vi "CRYAPI TAB.vi"(8 "tPage":T1, 9 "tFrame":T3, 10 "nData":i32, 11 "sAction":string) -> (0 "nData_Out":i32, 2 "tFrame_Out":T3, 3 "tPage_Out":T1)   [LabVIEW 2013]
uses:
  <vilib>/Utility/miscctls.llb/LVRectTypeDef.ctl
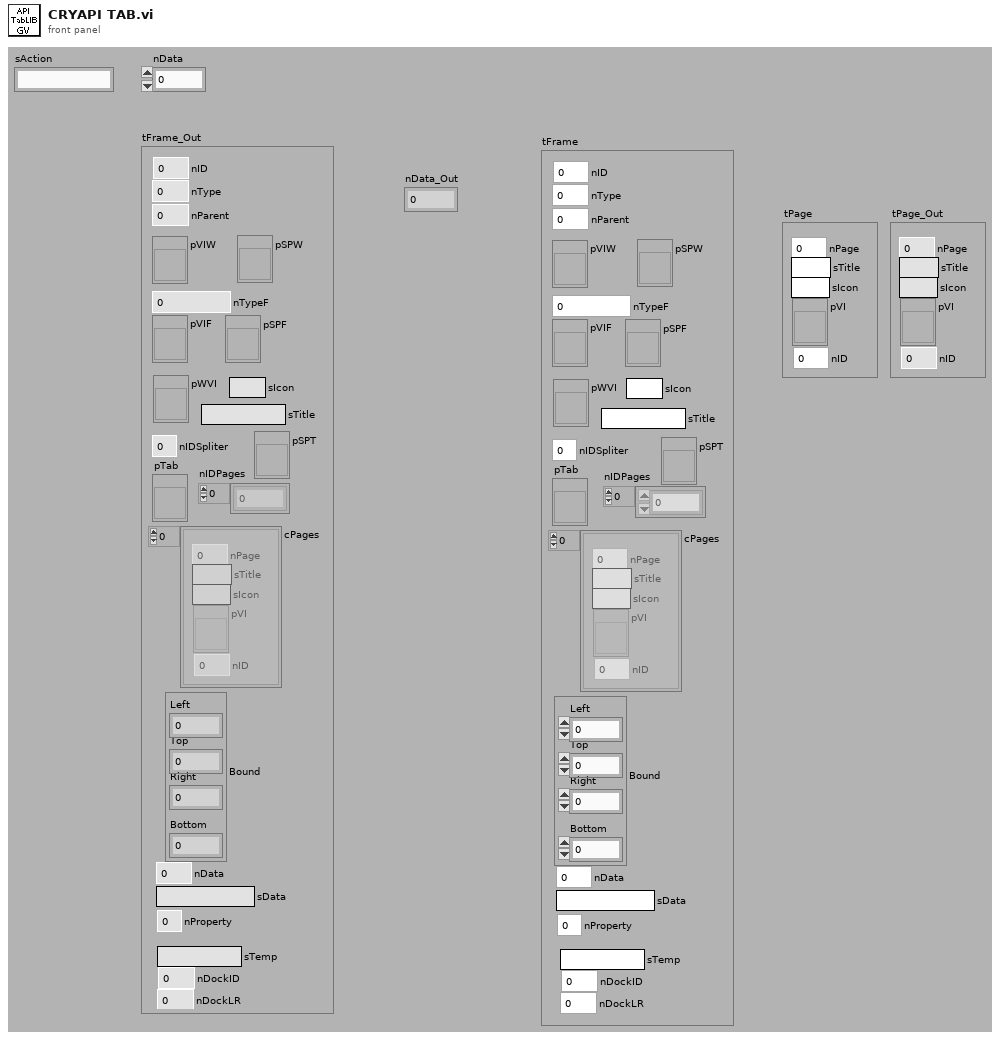
[diagram p1: front panel]
types:
  T1 = cluster{"nPage":i32, "sTitle":string, "sIcon":string, "pVI":refnum<vi>, "nID":i32}
  T2 = typedef "LVRectTypeDef.ctl" = cluster{"Left":i16, "Top":i16, "Right":i16, "Bottom":i16}
  T3 = cluster{"nType":i32, "nParent":i32, "pVIW":refnum<vi>, "pSPW":refnum<vi>, "nTypeF":i32, "pVIF":refnum<vi>, "pSPF":refnum<vi>, "nIDSpliter":i32, "nProperty":i32, "Bound":T2, "nID":i32, "nData":i32, "sData":string, "pWVI":refnum<vi>, "sTitle":string, "cPages":cluster{"nPage":i32, "sTitle":string, "sIcon":string, "pVI":refnum<vi>, "nID":i32}[], "pTab":refnum<vi>, "nIDPages":i32[], "pSPT":refnum<vi>, "sTemp":string, "nDockID":i32, "nDockLR":i32, "sIcon":string}
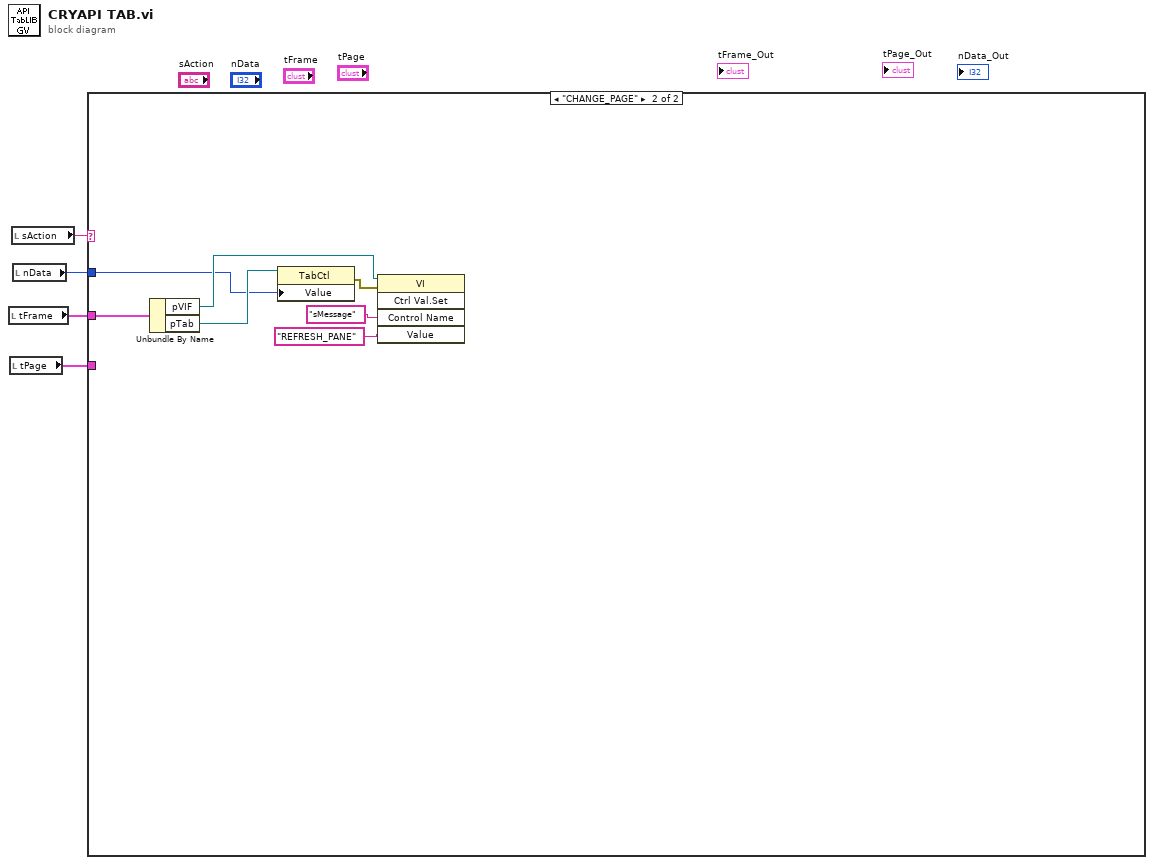
[diagram p0: block diagram]
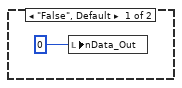
[diagram p2: hidden frame]
diagram:
  n1 = local read "tFrame"() -> (w3:T3)
  n2 = local read "tPage"() -> (w2:T1)
  n3 = local read "sAction"() -> (w4:string)
  n4 = local read "nData"() -> (w1:i32)
  n5 = case shown="\"CHANGE_PAGE\"" w4 {
    tunnel: w3 -> [_ w9]
    tunnel: w2 -> [_ _]
    tunnel: w1 -> [_ w6]
    frame "False", Default {
      n6 = local write "nData_Out"(0 ("nData_Out")) -> ()
    }
    frame "CHANGE_PAGE" {
      n7 = Unbundle By Name(w9) -> ("pVIF"=w8:refnum<vi>, "pTab"=w7:refnum<vi>)
      n8 = property class="TabCtl"(reference=w7, "Value"=w6) -> (error out=w10:errorcluster)  [unwired: 1 in, 1 out]
      n9 = invoke class="VI" method="Ctrl Val.Set"(reference=w8, error in=w10, "Control Name"="sMessage", "Value"="REFRESH_PANE" ("sAction")) -> ()  [unwired: 1 in, 5 out]
    }
  }
